vi "Unlock.vi"(0 "Interface_object in":refnum<class "Timed Door.lvclass">, 5 "error in (no error)":errorcluster) -> (14 "Interface_object out":refnum<class "Timed Door.lvclass">, 19 "error out":errorcluster)   [LabVIEW 2018, in "Timed Door.lvclass"]
uses:
  Timed Door.lvclass
  Timer/Timer.lvclass
  Timed Door.lvclass/Timed Door.ctl
  Timer/Timer.lvclass/Timer.ctl
  Get Door.vi
  Set Door.vi
  Timer/Get Target Time Elapsed Event.vi
  Set Timer DVR.vi
  Set Target Time Elapsed Event.vi
  Set Alarm DVR.vi
  Door/Door.lvclass
  Alarm/Alarm.lvclass
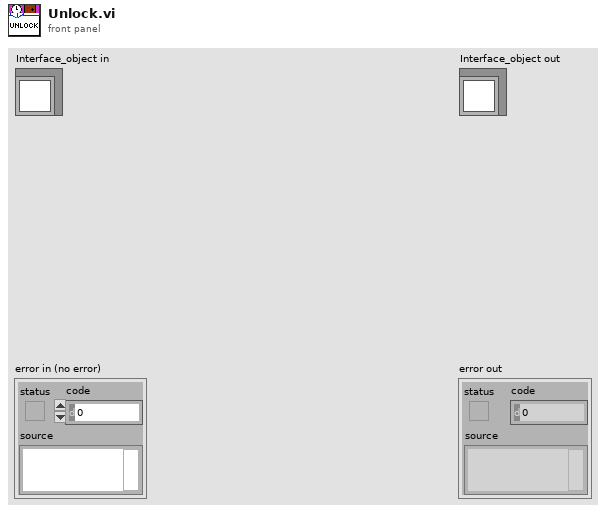
[diagram p1: front panel]
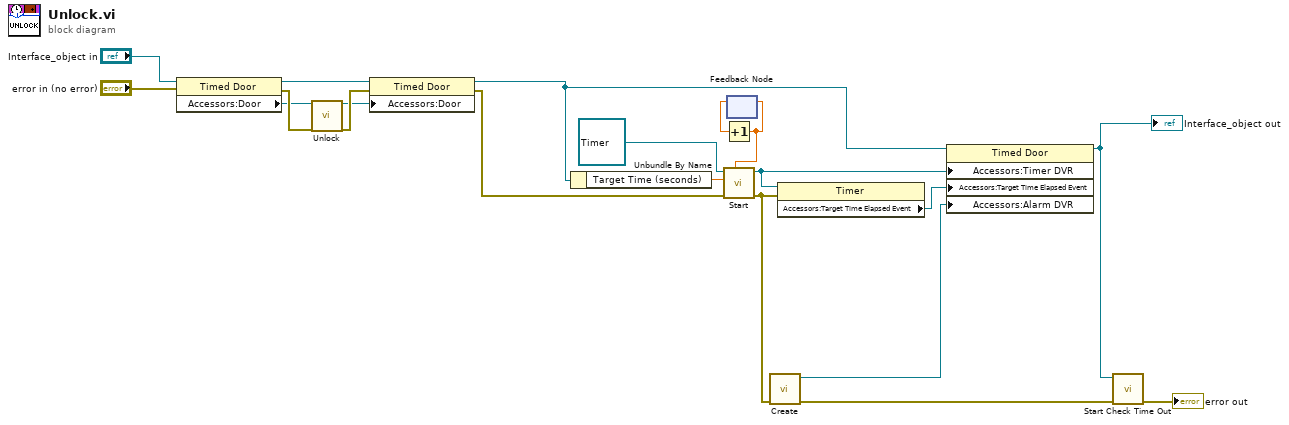
[diagram p0: block diagram]
diagram:
  n1 = property class="Timed Door"(reference="Interface_object in", error in="error in (no error)") -> (reference out=w19:refnum<class "Timed Door.lvclass">, error out=w17:errorcluster, "Accessors:Door"=w15:refnum<class "Door.lvclass">)
  n2 = call-dynamic "Unlock.vi"("Interface_object in"=w15, "error in (no error)"=w17) -> ("Interface_object out"=w14:refnum<class "Door.lvclass">, "error out"=w16:errorcluster)  [unwired: 16 in]
  n3 = property class="Timed Door"(reference=w19, error in=w16, "Accessors:Door"=w14) -> (reference out=w4:refnum<class "Timed Door.lvclass">, error out=w3:errorcluster)
  n4 = Unbundle By Name(w4) -> ("Target Time (seconds)"=w13:dbl)
  n5 = feedback #1() -> (w6:dbl)  [unwired: 1 in]
  n6 = Increment(x=w6) -> (x+1=w5:dbl)
  n7 = call-dynamic "Start.vi"("Timer ID"=w5, "error in (no error)"=w3, "Target Time (seconds)"=w13, "Timer in"=refnum<class "Timer.lvclass"> refnum) -> ("error out"=w9:errorcluster, "Timer DVR"=w8:refnum<data-value>)  [unwired: 6 in]
  n8 = feedback-in #1(w5) -> ()
  n9 = call "Create.vi"("error in (no error)"=w9) -> ("error out"=w10:errorcluster, "Alarm DVR"=w11:refnum<data-value>)  [unwired: 9 in]
  n10 = property class="Timer"(reference=w8, error in=w9) -> ("Accessors:Target Time Elapsed Event"=w7:refnum<user-event>)  [unwired: 2 out]
  n11 = property class="Timed Door"(reference=w4, "Accessors:Timer DVR"=w8, "Accessors:Target Time Elapsed Event"=w7, "Accessors:Alarm DVR"=w11) -> (reference out=w2:refnum<class "Timed Door.lvclass">)  [unwired: 1 in, 1 out]
  "Interface_object out" <- w2
  n12 = call "Start Check Time Out.vi"("error in (no error)"=w10, "Timed Door in"=w2) -> ("error out"=→"error out":errorcluster)  [unwired: 9 in]
